vi "CO Serial CAL & Data Recording & DECADEv4.1.vi"() -> ()   [LabVIEW 2014]
uses:
  <vilib>/Platform/TimedLoop/XDataNode/timing_clust.ctl
  <vilib>/Platform/TimedLoop/XDataNode/nitl_modes.ctl
  <vilib>/Platform/TimedLoop/XDataNode/wakeup.ctl
  C:/Program Files (x86)/National Instruments/LabVIEW 2014/examples/Data Communication/Network Streams/Simple Network Streams/support/Network Stream Command.ctl
  <vilib>/Utility/error.llb/whitespace.ctl
  <vilib>/Instr/_visa.llb/VISA Configure Serial Port (Instr).vi
  <vilib>/Utility/tcp.llb/UDP Multicast Write-Only Open.vi
  <vilib>/platform/TimedLoop/XDataNode/XDataNode.xnode
  <vilib>/Platform/TimedLoop/XDataNode/XDNodeRunTimeDep.lvlib
panel:
  out "Stop File Write":bool
  out "Default file name":string
  in  "Flight Number 2":string="XXXX"
  out "status":bool
  out "CO Vacuum":bool
  out "CO CAL":bool
  out "error out":errorcluster
  out "CO Vacuum?":i16
  out "Control data":i32[](array[numeric])
  out "Control data out":string
  in  "VISA resource name":refnum<visa-resource-name>="ASRL8::INSTR"
  out "Serial VISA error":errorcluster
  out "SEPTIC TCP Error Out":errorcluster
  out "TCP packet\nSend To SEPTIC":bool
  in  "msec to wait":u32=330 caption="mSec to Wait"
  out "UDP Time Stamp Offset":i32=1
  out "Scan from String Error \nCounter from process loop":i32
  out "TCP Binary Packet":string
  in  "ue9LJ temp":u16
  out "FISH TCP Error Out":errorcluster
  out "TCP packet\nSend To FISH":bool
  out "UDP_Out_Error Out":errorcluster
  out "Data Array":string[](array[string])
  out "UDP_Out Status":bool
  out "Data Process Status":bool
  out "Command In":string[](array[string])
  out "ERR Counter":i32
  out "UDP_Out":string
  out "UDP_Pack_num":u32
  out "Flight Number":string
  out "OK RAW COUNTER":i32
  out "IN_CAL?":bool
  out "Redundent DATA":string
  out "Data String":string
  out "CO_Data_Buffer":string[](array[string])
  out "RAW DATA":string
  out "loop count":i32
  out "Number of Read error":i32
  out "Command In":string
  # "Pre-flight"
  # "CONC"
  # "SIG"
  # "SENS"
  # "ZERO"
  # "Lamp flow controller"
  # "Lamp temperature"
  # "Monochromater flow controller"
  # "Monochromater temperature"
  # "Monochromater pressure"
  # "Fluorescence cell pressure"
  # "Calibration gas pressure"
  # "Cell temperature"
  # "Calibration Concentration"
  # "ERROR number"
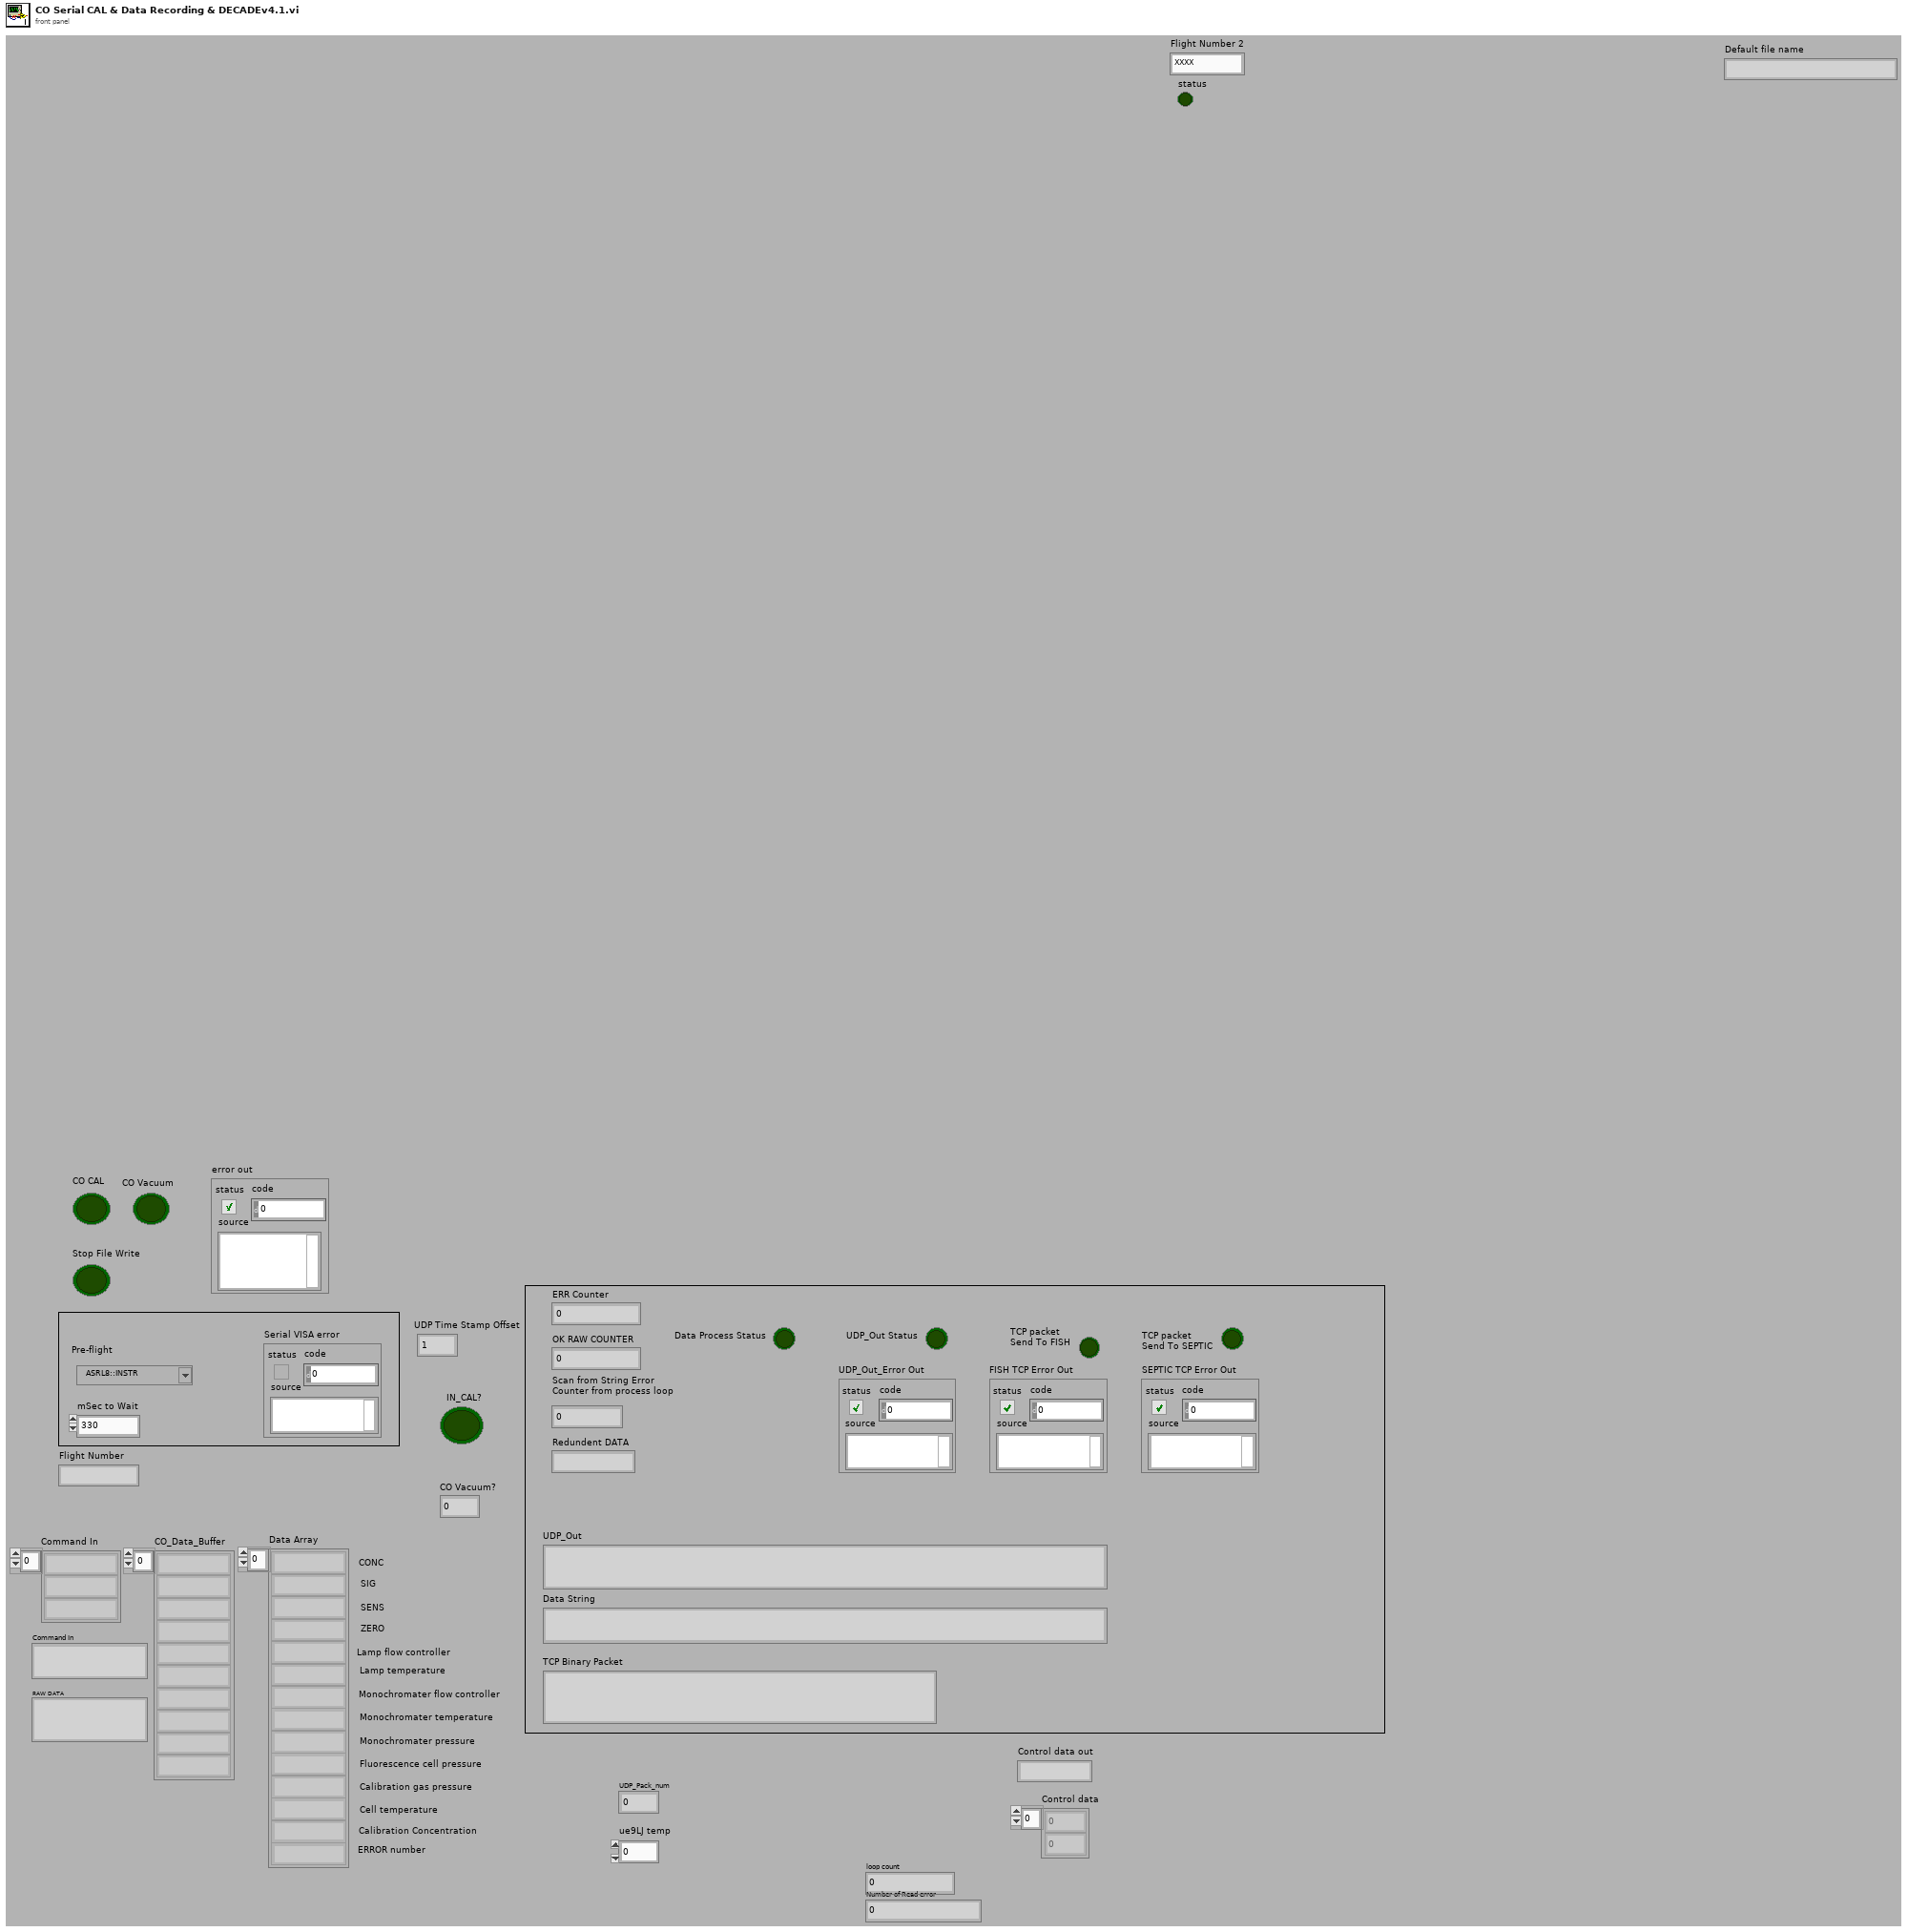
[diagram p1: front panel]
types:
  T1 = typedef "XDNodeRunTimeDep.lvlib/timing_clust.ctl" = cluster{"Expected End [f-1]":u64, "Actual End [f-1]":u64, "Finished Late? [f-1]":bool, "Expected End [i-1]":u64, "Actual End [i-1]":u64, "Finished Late? [i-1]":bool, "Expected Start [i]":u64, "Actual Start [i]":u64, "Expected Start [f]":u64, "Actual Start [f]":u64, "Source Name":string, "Structure Name":string, "Period":i64, "Deadline":i64, "Offset":i64, "Start":i64, "Priority":i32, "Timeout":i32, "Mode":T2, "Wakeup Reason":T3, "Error":errorcluster, "Source Type":string, "Secondary Source Type":string, "Global End Time":u64, "Global Start Time":u64, "Frame Duration":u64, "Iteration Duration":u64, "Assigned CPU":i32, "I/O Scan Engine Mode":u32}
  T2 = typedef "XDNodeRunTimeDep.lvlib/nitl_modes.ctl" = enum32{"No Change", "Process missed periods, maintain original phase", "Discard missed periods, maintain original phase", "Process missed periods, ignore original phase", "Discard missed periods, ignore original phase"}
  T3 = typedef "XDNodeRunTimeDep.lvlib/wakeup.ctl" = enum32{"Normal", "Aborted", "Asynchronous wakeup", "Timing source error", "Timed loop error", "Timeout"}
  T4 = typedef "Network Stream Command.ctl" = cluster{"Message":string, "Message Data":variant}
  T5 = enum16{"open", "replace", "create", "open or create", "replace or create", "replace or create with confirmation"}
  T6 = typedef "whitespace.ctl" = u16
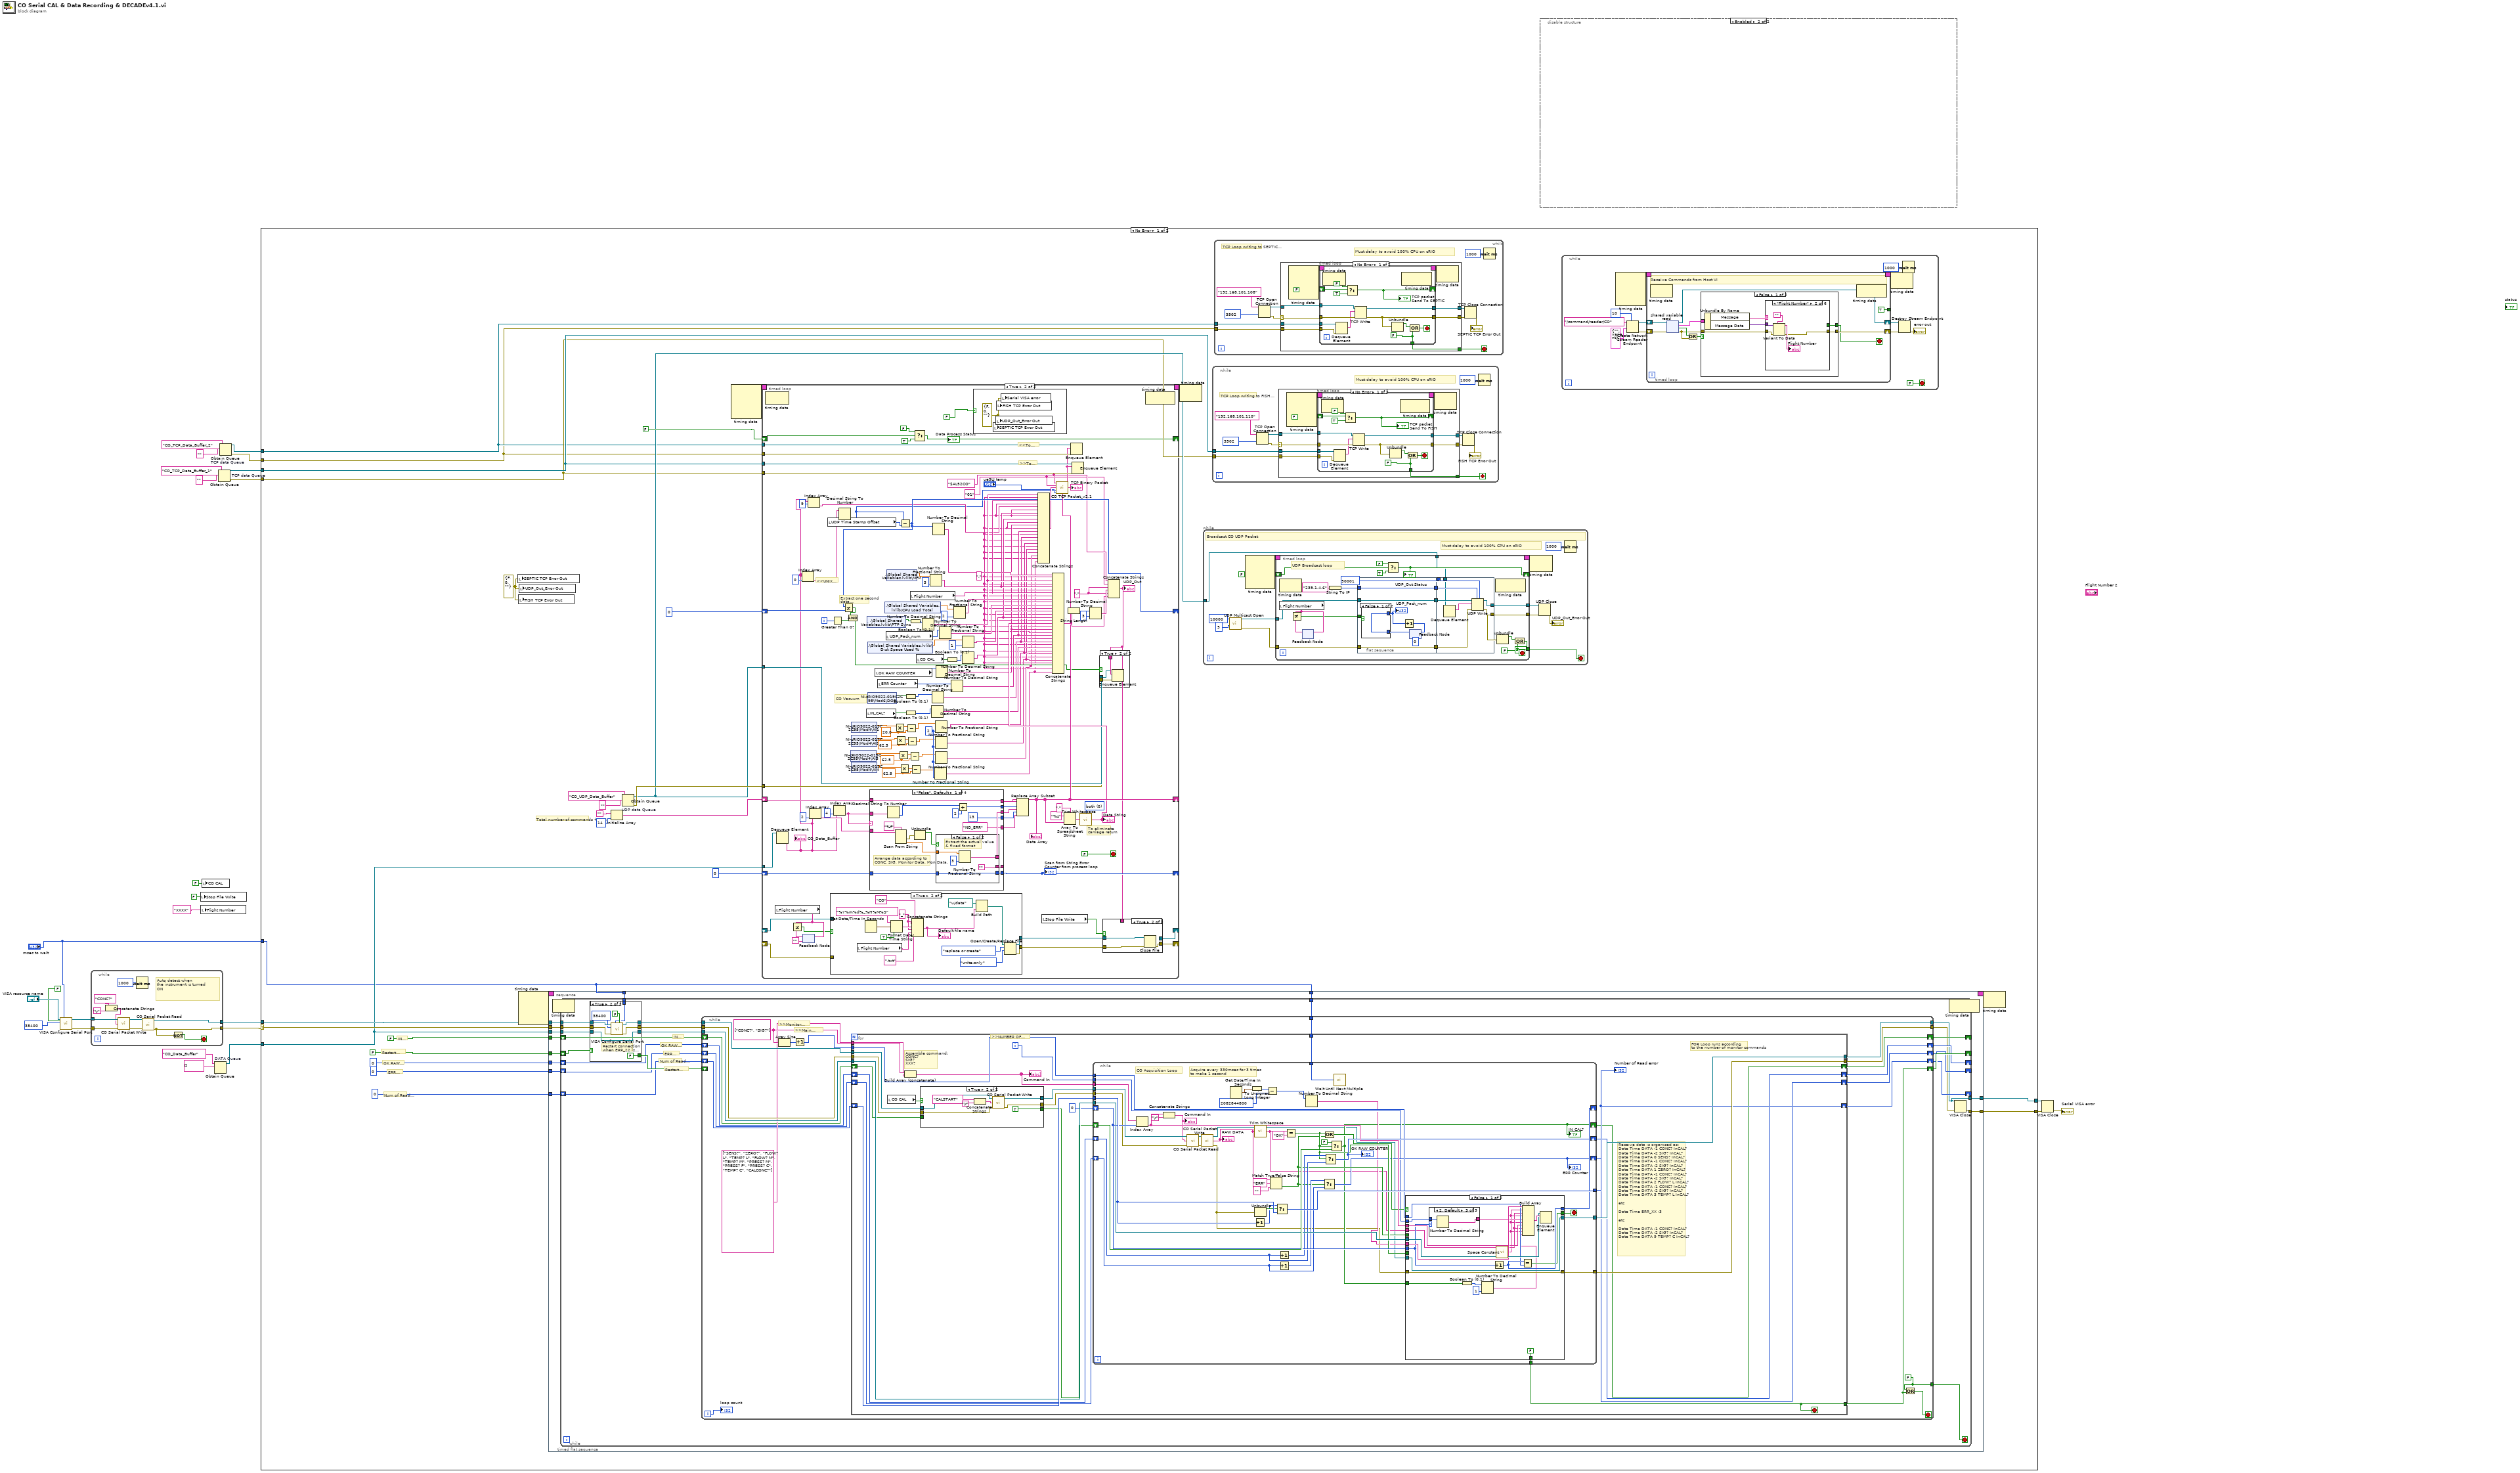
[diagram p0: block diagram]
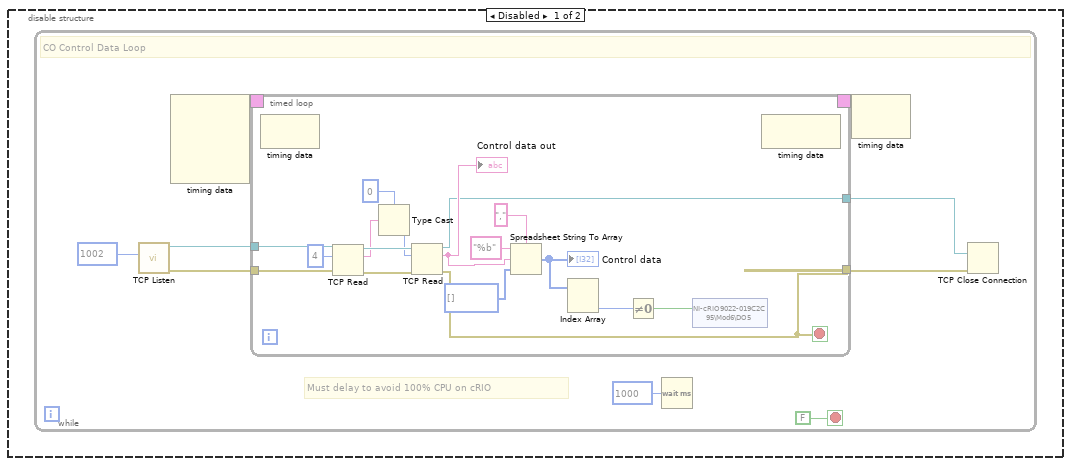
[diagram p2: hidden frame]
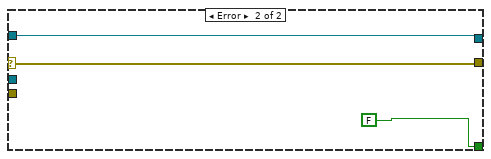
[diagram p3: hidden frame]
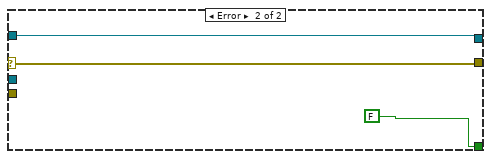
[diagram p4: hidden frame]
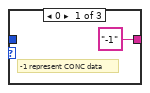
[diagram p6: hidden frame]
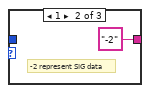
[diagram p7: hidden frame]
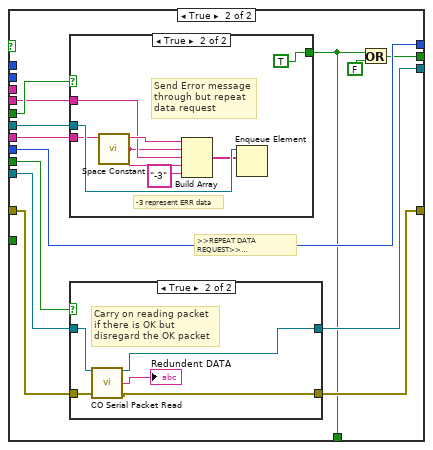
[diagram p8: hidden frame]
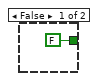
[diagram p10: hidden frame]
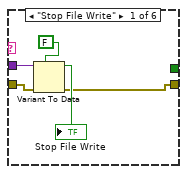
[diagram p12: hidden frame]
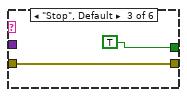
[diagram p13: hidden frame]
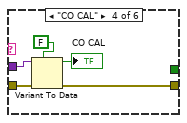
[diagram p14: hidden frame]
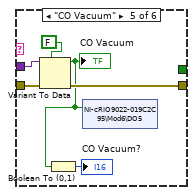
[diagram p15: hidden frame]
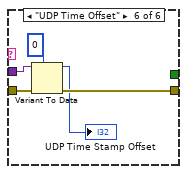
[diagram p16: hidden frame]
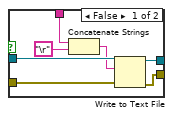
[diagram p19: hidden frame]
diagram:
  n1 = call-poly "VISA Configure Serial Port"("VISA resource name"="VISA resource name", "timeout (10sec)"="msec to wait", "Enable Termination\nChar (T)"=FALSE ("Enable Termination\nChar (T)"), "baud rate (9600)"=u32 38400) -> ("VISA resource name out"=w12:refnum<visa-resource-name>, "error out"=w11:errorcluster)  [unwired: 10 in]
  n2 = while {
    tunnel: w12 -> [w36]
    tunnel: w11 -> [w35]
    tunnel: [w29] -> w10
    tunnel: [w30] -> w9
    stop <- w34 stop-if-true
    # "Auto detect when\nthe instrument is turned \nON"
    n3 = Concatenate Strings("CONC?" ("Data in"), "\r") -> (w26:string)
    n4 = call "CO Serial Packet Write.vi"("VISA resource name In"=w36, "Data in"=w26, "error in (no error)"=w35) -> ("VISA resource name Out"=w32:refnum<visa-resource-name>, "error out"=w31:errorcluster)  [unwired: 11 in]
    n5 = Wait (ms)(milliseconds to wait=u32 1000) -> ()  [unwired: 1 out]
    n6 = call "CO Serial Packet Read.vi"("VISA resource In"=w32, "error in"=w31) -> ("VISA resource Out"=w29:refnum<visa-resource-name>, "error out"=w30:errorcluster)  [unwired: 11 in, 1 out]
    n7 = Not(x=w30) -> (.not. x?=w34:bool)
  }
  n8 = local write "Stop File Write"(FALSE ("Stop File Write")) -> ()
  n9 = local write "Flight Number"("XXXX" ("Flight Number")) -> ()
  n10 = local write "CO CAL"(FALSE ("CO CAL")) -> ()
  n11 = Obtain Queue "DATA Queue"(name (unnamed)="CO_Data_Buffer", element data type=string[] []) -> (queue out=w23:refnum<queue>)  [unwired: 3 in, 2 out]
  n12 = Obtain Queue "TCP data Queue"(name (unnamed)="CO_TCP_Data_Buffer_1", element data type="") -> (queue out=w22:refnum<queue>, error out=w21:errorcluster)  [unwired: 3 in, 1 out]
  n13 = Obtain Queue "TCP data Queue"(name (unnamed)="CO_TCP_Data_Buffer_2", element data type="") -> (queue out=w20:refnum<queue>, error out=w19:errorcluster)  [unwired: 3 in, 1 out]
  n14 = case shown="No Error" w9 {
    selector: w9 -> [w64 w715]
    tunnel: w10 -> [w65 w714]
    tunnel: [w66 w715] -> w15
    tunnel: [w42 w714] -> w14
    tunnel: w23 -> [w63 _]
    tunnel: w22 -> [w52 _]
    tunnel: w21 -> [w51 _]
    tunnel: w20 -> [w50 _]
    tunnel: w19 -> [w49 _]
    tunnel: "msec to wait" -> [w37 _]
    frame No Error {
      w48 = errorcluster {"status"=FALSE, "code"=0, "source"=""} ("UDP_Out_Error Out")
      # "Restart connection?"
      # "IN CAL?"
      # "OK RAW Counter"
      # "ERR Counter"
      # "Num of Read Error"
      # "Total number of commands + ERR"
      n15 = local write "SEPTIC TCP Error Out"(w48) -> ()
      n16 = node-c288() -> (w39:T1)  [unwired: 4 in]
      n17 = local write "FISH TCP Error Out"(w48) -> ()
      n18 = local write "UDP_Out_Error Out"(w48) -> ()
      n19 = timed-sequence {
        timing: w39 -> [_]
        timing-out: [_] -> w38
        tunnel: [w162] -> w66
        tunnel: w65 -> [w161]
        tunnel: w64 -> [w160]
        tunnel: w63 -> [w159]
        tunnel: FALSE -> [w158]
        tunnel: 0 -> [w157]
        tunnel: 0 -> [w156]
        tunnel: 0 -> [w155]
        tunnel: FALSE ("IN_CAL?") -> [w154]
        tunnel: [w153] -> w42
        tunnel: w37 -> [w152]
        tunnel: w37 -> [w151]
        n20 = timed-flat-sequence {
          tunnel: [w174] -> w162
          tunnel: w161 -> [w173]
          tunnel: w160 -> [w172]
          tunnel: w159 -> [w171]
          tunnel: w158 -> [w170]
          tunnel: w157 -> [w169]
          tunnel: w156 -> [w168]
          tunnel: w155 -> [w167]
          tunnel: w154 -> [w166]
          tunnel: [w165] -> w153
          tunnel: w152 -> [w164]
          tunnel: w151 -> [w163]
          n21 = node-c288() -> ()  [unwired: 1 in, 1 out]
          n22 = while {
            tunnel: [w179] -> w174
            tunnel: w173 -> [w196]
            tunnel: w172 -> [w195]
            tunnel: w171 -> [w193]
            shift-right: [w190] -> _
            shift-left: w170 -> [w191]
            shift-right: [w186] -> _
            shift-left: w169 -> [w187]
            shift-right: [w183] -> _
            shift-left: w168 -> [w185]
            shift-right: [w182] -> _
            shift-left: w167 -> [w184]
            shift-right: [w180] -> _
            shift-left: w166 -> [w181]
            tunnel: [w177] -> w165
            tunnel: w164 -> [w176]
            tunnel: w163 -> [w175]
            stop <- w189 stop-if-true
            # "Restart connection?"
            # "Num of Read Error"
            # "ERR Counter"
            # "IN CAL?"
            # "OK RAW Counter"
            n23 = case shown="True" w191 {
              selector: w191 -> [w198 _]
              tunnel: [w201 w207] -> w197
              tunnel: w196 -> [w201 w208]
              tunnel: [w200 w206] -> w194
              tunnel: w195 -> [w200 w205]
              tunnel: [w199 w210] -> w192
              tunnel: w193 -> [w199 w210]
              tunnel: [w198 FALSE] -> w188
              tunnel: w175 -> [_ w202]
              frame False {
              }
              frame True {
                # "Restart connection\nwhen ERR_22 is detected"
                n24 = call-poly "VISA Configure Serial Port"("VISA resource name"=w208, "timeout (10sec)"=w202, "Enable Termination\nChar (T)"=FALSE ("Enable Termination\nChar (T)"), "baud rate (9600)"=u32 38400, "error in (no error)"=w205) -> ("VISA resource name out"=w207:refnum<visa-resource-name>, "error out"=w206:errorcluster)  [unwired: 9 in]
              }
            }
            n25 = while {
              tunnel: [w232] -> w178
              tunnel: w197 -> [w231]
              tunnel: w194 -> [w230]
              tunnel: [w229] -> w177
              tunnel: w192 -> [w228]
              shift-right: [w219] -> w186
              shift-left: w187 -> [w223]
              shift-right: [w218] -> w183
              shift-left: w185 -> [w222]
              shift-right: [w217] -> w180
              shift-left: w181 -> [w221]
              shift-right: [w216] -> w182
              shift-left: w184 -> [w220]
              tunnel: [w212] -> w189
              shift-right: [w213] -> w190
              shift-left: w188 -> [_]
              tunnel: w176 -> [w211]
              i -> [w215]
              stop <- w214 stop-if-true
              w212 = FALSE
              w227 = string[] ["CONC?", "SIG?"]
              # ">>Main commands>>"
              # ">>Monitor Command>>"
              n26 = Array Size(array=w227) -> (size(s)=w224:i32)
              n27 = Increment(x=w224) -> (x+1=w226:i32)
              n28 = for {
                tunnel: w231 -> [w252]
                tunnel: w230 -> [w251]
                tunnel: [w257] -> w232
                shift-right: [w255] -> w216
                shift-left: w220 -> [w256]
                tunnel: [w254] -> w229
                tunnel: w228 -> [w253]
                tunnel: w226 -> [w247]
                shift-right: [w245] -> w217
                shift-left: w221 -> [w246]
                shift-right: [w243] -> w218
                shift-left: w222 -> [w244]
                shift-right: [w241] -> w219
                shift-left: w223 -> [w242]
                tunnel: string[] ["SENS?", "ZERO?", "FLOW? L", "TEMP? L", "FLOW? M", "TEMP? M", "PRESS? M", "PRESS? F", "PRESS? C", "TEMP? C", "CALCONC?"] -> [w238] mode=indexing
                tunnel: w227 -> [w239]
                tunnel: [w236] -> w213
                tunnel: w211 -> [w234]
                i -> [w237]
                stop <- w236 stop-if-true
                # "Receive data is organised as:\nDate Time DATA -1 CONC? InCAL?\nDate Time DATA -2 SIG? InCAL?\nDate Time DATA 0 SENS? InCAL?\nDate Time DATA -1 CONC? InCAL?\nDate Time DATA -2 SIG? InCAL?\nDate Time DATA 1 ZERO? InCAL?\nDate Time DATA -1 CONC? InCAL?\nDate Time DATA -2 SIG? InCAL?\nDate Time DATA 2 FLOW? L InCAL?\nDate Time DATA -1 CONC? InCAL?\nDate Time DATA -2 SIG? InCAL?\nDate Time DATA 3 TEMP? L InCAL?\n\netc\n\nDate Time ERR_XX -3\n\netc\n\nDate Time DATA -1 CONC? InCAL?\nDate Time DATA -2 SIG? InCAL?\nDate Time DATA 9 TEMP? C InCAL?"
                # "FOR Loop runs according\nto the number of monitor commands"
                # "Assemble command:\nCONC?\nSIG?\nXXX?"
                # ">>NUMBER OF COMMANDS>>"
                n29 = local read "CO CAL"() -> (w233:bool)
                n30 = Build Array (concatenate)(w239, w238) -> (w240:string[])
                "Command In" <- w240
                n31 = case shown="True" w233 {
                  tunnel: w252 -> [w357 w359]
                  tunnel: w251 -> [w356 w362]
                  tunnel: [w357 w360] -> w250
                  tunnel: [w356 w361] -> w249
                  tunnel: [w355 TRUE ("IN_CAL?")] -> w248
                  tunnel: w246 -> [w355 _]
                  frame False {
                  }
                  frame True {
                    n32 = Concatenate Strings("CALSTART" ("string"), "\r") -> (w358:string)
                    n33 = call "CO Serial Packet Write.vi"("VISA resource name In"=w359, "Data in"=w358, "error in (no error)"=w362) -> ("VISA resource name Out"=w360:refnum<visa-resource-name>, "error out"=w361:errorcluster)  [unwired: 11 in]
                  }
                }
                n34 = while {
                  tunnel: w249 -> [w264]
                  tunnel: [w291] -> w257
                  tunnel: w256 -> [w303]
                  tunnel: [w302] -> w255
                  tunnel: w240 -> [w295]
                  tunnel: [w292] -> w254
                  tunnel: w253 -> [w290]
                  tunnel: w250 -> [w266]
                  shift-right: [w267] -> w245
                  shift-left: w248 -> [w297]
                  shift-right: [w294] -> _
                  shift-left: 0 -> [w296]
                  tunnel: w247 -> [w287]
                  shift-right: [w284] -> w243
                  shift-left: w244 -> [w285]
                  shift-right: [w278] -> w241
                  shift-left: w242 -> [w280]
                  tunnel: w237 -> [w277]
                  tunnel: [w272] -> w236
                  tunnel: w234 -> [w258]
                  stop <- w293 stop-if-true
                  # "Acquire every 330msec for 3 times\nto make 1 second"
                  # "CO Acquisition Loop"
                  n35 = Index Array(array=w295, index=w296) -> (element=w289:string)
                  n36 = Concatenate Strings(w289, "\r") -> (w265:string)
                  "Command In" <- w265
                  n37 = call "CO Serial Packet Write.vi"("VISA resource name In"=w266, "Data in"=w265, "error in (no error)"=w264) -> ("VISA resource name Out"=w262:refnum<visa-resource-name>, "error out"=w263:errorcluster)  [unwired: 11 in]
                  n38 = call "CO Serial Packet Read.vi"("VISA resource In"=w262, "error in"=w263) -> ("VISA resource Out"=w261:refnum<visa-resource-name>, "Data Out"=w259:string, "error out"=w260:errorcluster)  [unwired: 11 in]
                  "RAW DATA" <- w259
                  n39 = Get Date/Time In Seconds() -> (seconds since 1Jan1904=w273:timestamp)
                  n40 = To Unsigned Long Integer(number=w273) -> (unsigned 32bit integer=w276:u32)
                  n41 = Increment(x=w303) -> (x+1=w299:i32)
                  n42 = call <vilib>:"Trim Whitespace.vi"("string"=w259) -> ("trimmed string"=w271:string)  [unwired: 1 in]
                  n43 = Unbundle(w260) -> ("status"=w300:bool)  [unwired: 2 out]
                  n44 = Subtract(x=w276, y=u32 2082844800) -> (x-y=w268:u32)
                  n45 = Match True/False String(2:"" ("false string"), 3:"ERR" ("true string"), 4:w259) -> (0:w279:bool)  [unwired: 1 out]
                  n46 = Select(t=w299, s=w300, f=w303) -> (s? t:f=w302:i32)
                  n47 = Increment(x=w285) -> (x+1=w286:i32)
                  n48 = Increment(x=w280) -> (x+1=w281:i32)
                  n49 = Equal?(x=w271, y="OK" ("string")) -> (x = y?=w282:bool)
                  n50 = Number To Decimal String(number=w268) -> (decimal integer string=w274:string)  [unwired: 1 in]
                  n51 = Select(t=w281, s=w279, f=w280) -> (s? t:f=w278:i32)
                  "ERR Counter" <- w278
                  n52 = Select(t=w286, s=w282, f=w285) -> (s? t:f=w284:i32)
                  "OK RAW COUNTER" <- w284
                  n53 = Compound Arithmetic op=OR(w282, w279) -> (w283:bool)
                  n54 = Select(t=FALSE, s=w282, f=w297) -> (s? t:f=w267:bool)
                  "IN_CAL?" <- w267
                  n55 = call "Wait Until Next Multiple"("Count(mSec)"=w258) -> ()  [unwired: 1 out]
                  n56 = case shown="False" w283 {
                    tunnel: w296 -> [w311 w339]
                    tunnel: [w322 w339] -> w294
                    tunnel: [w316 w329] -> w293
                    tunnel: w261 -> [w321 w338]
                    tunnel: w260 -> [w320 w337]
                    tunnel: [w321 w336] -> w292
                    tunnel: [w320 w335] -> w291
                    tunnel: w290 -> [w318 w333]
                    tunnel: w271 -> [w309 w331]
                    tunnel: w289 -> [w312 _]
                    tunnel: w274 -> [w317 w332]
                    tunnel: w279 -> [_ w334]
                    tunnel: w287 -> [w315 _]
                    tunnel: w282 -> [_ w330]
                    tunnel: w277 -> [w314 _]
                    tunnel: [FALSE w327] -> w272
                    tunnel: w267 -> [w308 _]
                    frame False {
                      n57 = case shown="2, Default" w311 {
                        tunnel: w314 -> [_ _ w326]
                        tunnel: ["-1" "-2" w325] -> w313
                        frame 0 {
                          # "-1 represent CONC data"
                        }
                        frame 1 {
                          # "-2 represent SIG data"
                        }
                        frame 2, Default {
                          n58 = Number To Decimal String(number=w326) -> (decimal integer string=w325:string)  [unwired: 1 in]
                        }
                      }
                      n59 = Boolean To (0,1)(Boolean=w308) -> (0, 1=w307:i16)
                      n60 = Number To Decimal String(number=w307, width (-)=i16 1) -> (decimal integer string=w304:string)
                      n61 = Increment(x=w311) -> (x+1=w322:i32)
                      n62 = call <vilib>:"Space Constant.vi"() -> ("String"=w305:string)
                      n63 = Equal?(x=w322, y=w315) -> (x = y?=w316:bool)
                      n64 = Build Array(w317, w305, w309, w305, w313, w305, w312, w309, w305, w304) -> (w319:string[])
                      n65 = Enqueue Element(queue=w318, element=w319) -> ()  [unwired: 2 in, 3 out]
                    }
                    frame True {
                      # ">>REPEAT DATA REQUEST>>\nif OK or ERR"
                      n66 = case shown="True" w334 {
                        tunnel: w333 -> [_ w354]
                        tunnel: w332 -> [_ w352]
                        tunnel: w331 -> [_ w351]
                        tunnel: [FALSE TRUE] -> w327
                        frame False {
                        }
                        frame True {
                          # "-3 represent ERR data"
                          # "Send Error message\nthrough but repeat\ndata request"
                          n67 = call <vilib>:"Space Constant.vi"() -> ("String"=w350:string)
                          n68 = Build Array(w352, w350, w351, w350, "-3" ("element")) -> (w353:string[])
                          n69 = Enqueue Element(queue=w354, element=w353) -> ()  [unwired: 2 in, 3 out]
                        }
                      }
                      n70 = case shown="True" w330 {
                        tunnel: w338 -> [w340 w345]
                        tunnel: w337 -> [w341 w346]
                        tunnel: [w340 w344] -> w336
                        tunnel: [w341 w342] -> w335
                        frame False {
                        }
                        frame True {
                          # "Carry on reading packet\nif there is OK but\ndisregard the OK packet"
                          n71 = call "CO Serial Packet Read.vi"("VISA resource In"=w345, "error in"=w346) -> ("VISA resource Out"=w344:refnum<visa-resource-name>, "Data Out"=→"Redundent DATA":string, "error out"=w342:errorcluster)  [unwired: 11 in]
                        }
                      }
                      n72 = Or(x=w327, y=FALSE) -> (x .or. y?=w329:bool)
                    }
                  }
                }
                "Number of Read error" <- w255
              }
              n73 = Or(x=w212, y=w213) -> (x .or. y?=w214:bool)
              "loop count" <- w215
            }
            n74 = VISA Close(VISA resource name=w177, error in (no error)=w178) -> (error out=w179:errorcluster)
          }
          n75 = node-c288() -> ()  [unwired: 1 in, 1 out]
        }
      }
      n76 = Initialize Array("", 14) -> (w60:string[])
      n77 = Obtain Queue "UDP data Queue"(name (unnamed)="CO_UDP_Data_Buffer", element data type="") -> (queue out=w55:refnum<queue>, error out=w56:errorcluster)  [unwired: 3 in, 1 out]
      n78 = node-c288() -> (w41:T1)  [unwired: 4 in]
      n79 = timed-loop {
        tunnel: w63 -> [w548]
        shift-right: [w523] -> _
        shift-left: w60 -> [w537]
        shift-right: [w524] -> _
        shift-left: FALSE -> [w527]
        tunnel: w52 -> [w522]
        tunnel: w51 -> [w521]
        tunnel: w55 -> [w519]
        tunnel: w56 -> [w518]
        shift-right: [w516] -> _
        shift-left: 0 -> [w517]
        shift-right: [w504] -> _
        shift-left: 0 -> [w510]
        tunnel: w50 -> [w508]
        tunnel: w49 -> [w507]
        timing: w41 -> [_]
        timing-out: [_] -> w40
        shift-right: [w495] -> _
        shift-left: _ -> [w488]
        shift-right: [w486] -> _
        shift-left: _ -> [w487]
        i -> [w513]
        stop <- FALSE stop-if-true
        w469 = 62.5 ("y")
        w470 = 62.5 ("y")
        w473 = 62.5 ("y")
        w476 = 20.0 ("y")
        w498 = i16 2 ("precision (6)")
        w529 = T6 0 items=["both", "start of string", "end of string"] ("location (both)")
        w438 = ","
        w434 = "01"
        w540 = ","
        w435 = "$AL52CO"
        # "CO Vacuum"
        # ">>To SEPTIC>>"
        # ">>To FISH>>"
        # "Extract one second data\nfor UDP sending"
        # ">>UNIX TIME>>"
        # "To eliminate\ncarriage return"
        n80 = node-c288() -> ()  [unwired: 1 in, 1 out]
        n81 = local read "Flight Number"() -> (w493:string)
        n82 = Dequeue Element(queue=w548) -> (element=w500:string[])  [unwired: 2 in, 3 out]
        "CO_Data_Buffer" <- w500
        n83 = Index Array(array=w500, index=0) -> (element=w511:string)
        n84 = feedback #1("" ("Flight Number")) -> (w492:string)
        n85 = Not Equal?(x=w493, y=w492) -> (x != y?=w491:bool)
        n86 = feedback-in #1(w493) -> ()
        n87 = Index Array(array=w500, index=9) -> (element=w447:string)
        n88 = Index Array(array=w500, index=2) -> (element=w535:string)
        n89 = local read "UDP Time Stamp Offset"() -> (w450:i32)
        n90 = case shown="True" w491 {
          tunnel: [w550 w552] -> w490
          tunnel: [w549 w551] -> w489
          tunnel: w488 -> [w550 _]
          tunnel: w487 -> [w549 _]
          frame False {
          }
          frame True {
            w559 = "_" ("string")
            n91 = local read "Flight Number"() -> (w565:string)
            n92 = Get Date/Time In Seconds() -> (seconds since 1Jan1904=w560:timestamp)
            n93 = Format Date/Time String(time format string (%c)="%Y%m%d%_%H%M%S", seconds (now)=w560, UTC format=TRUE) -> (date/time string=w563:string)
            n94 = Concatenate Strings("CO" ("string"), w559, w563, w559, w565, ".txt" ("string")) -> (w557:string)
            "Default file name" <- w557
            n95 = Build Path(base path=path "u:/data", name or relative path=w557) -> (appended path=w553:path)
            n96 = Open/Create/Replace File(file path (use dialog)=w553, operation (0:open)=T5."replace or create", access (0:read/write)=enum16{"read/write", "read-only", "write-only"}."write-only") -> (refnum out=w552:refnum<file>, error out=w551:errorcluster)  [unwired: 3 in, 1 out]
          }
        }
        n97 = Greater Than 0?(x=w513) -> (x > 0?=w512:bool)
        n98 = Index Array(array=w500, index=4) -> (element=w536:string)
        n99 = Decimal String To Number(string=w511) -> (number=w433:i32)  [unwired: 2 in, 1 out]
        n100 = shared-variable "NI-cRIO9022-019C2C95\\Mod4\\AI3"() -> (w468:dbl)  [unwired: 1 in, 1 out]
        n101 = shared-variable "NI-cRIO9022-019C2C95\\Mod4\\AI4"() -> (w466:dbl)  [unwired: 1 in, 1 out]
        n102 = shared-variable "NI-cRIO9022-019C2C95\\Mod4\\AI1"() -> (w478:dbl)  [unwired: 1 in, 1 out]
        n103 = shared-variable "NI-cRIO9022-019C2C95\\Mod4\\AI2"() -> (w472:dbl)  [unwired: 1 in, 1 out]
        n104 = local read "IN_CAL?"() -> (w455:bool)
        n105 = shared-variable ".\\Global Shared Variables.lvlib\\PTP Sync"() -> (w479:bool)  [unwired: 1 in, 1 out]
        n106 = shared-variable ".\\Global Shared Variables.lvlib\\Disk Space Used %"() -> (w459:dbl)  [unwired: 1 in, 1 out]
        n107 = shared-variable "NI-cRIO9022-019C2C95\\Mod6\\DO5"() -> (w452:bool)  [unwired: 1 in, 1 out]
        n108 = case shown="\"False\", Default" w536 {
          tunnel: w536 -> [w596 _ _ _]
          tunnel: w537 -> [w597 w619 w641 w655]
          tunnel: w535 -> [w588 w613 w635 w651]
          tunnel: [w597 w619 w641 w655] -> w534
          tunnel: [w594 0 ("index") 1 ("index") w652] -> w533
          tunnel: [w587 w609 w631 w651] -> w532
          tunnel: [w586 w610 w632 ""] -> _
          tunnel: w517 -> [w585 w612 w634 w653]
          tunnel: [w584 w611 w633 w653] -> w516
          tunnel: [13 ("index") 13 ("index") 13 ("index") w652] -> w503
          tunnel: ["NO_ERR" "NO_ERR" "NO_ERR" w651] -> w502
          frame "False", Default {
            # "Arrange data according to\nCONC, SIG, Monitor Data, Mon Data,"
            n109 = Decimal String To Number(string=w596) -> (number=w593:i32)  [unwired: 2 in, 1 out]
            n110 = Scan From String(format string="%f", input string=w588) -> (error out=w590:errorcluster, output 1=w591:dbl)  [unwired: 3 in, 2 out]
            n111 = Unbundle(w590) -> ("status"=w589:bool)  [unwired: 2 out]
            n112 = case shown="False" w589 {
              tunnel: [w602 ""] -> w587
              tunnel: w591 -> [w601 _]
              tunnel: w585 -> [w600 w605]
              tunnel: [w600 w604] -> w584
              tunnel: ["" "Scan from string error"] -> w586
              frame False {
                # "Extract the actual value\n& fixed format"
                n113 = Number To Fractional String(number=w601, precision (6)=i16 3) -> (F-format string=w602:string)  [unwired: 2 in]
              }
              frame True {
                # "If scan from string error,\nreplace data with empty\nstring"
                n114 = Increment(x=w605) -> (x+1=w604:i32)
              }
            }
            n115 = Add(x=w593, y=2) -> (x+y=w594:i32)
          }
          frame "-1" {
            # "Arrange data according to\nCONC, SIG, Monitor Data, Mon Data,"
            # "-1 represent CONC data"
            n116 = Scan From String(format string="%f", input string=w613) -> (error out=w615:errorcluster, output 1=w616:dbl)  [unwired: 3 in, 2 out]
            n117 = Unbundle(w615) -> ("status"=w614:bool)  [unwired: 2 out]
            n118 = case shown="False" w614 {
              tunnel: [w624 ""] -> w609
              tunnel: w616 -> [w623 _]
              tunnel: w612 -> [w622 w627]
              tunnel: [w622 w626] -> w611
              tunnel: ["" "Scan from string error"] -> w610
              frame False {
                # "Extract the actual value\n& fixed format"
                n119 = Number To Fractional String(number=w623, precision (6)=i16 5) -> (F-format string=w624:string)  [unwired: 2 in]
              }
              frame True {
                # "If scan from string error,\nreplace data with empty\nstring"
                n120 = Increment(x=w627) -> (x+1=w626:i32)
              }
            }
          }
          frame "-2" {
            # "Arrange data according to\nCONC, SIG, Monitor Data, Mon Data,"
            # "-2 represent SIG data"
            n121 = Scan From String(format string="%f", input string=w635) -> (error out=w637:errorcluster, output 1=w638:dbl)  [unwired: 3 in, 2 out]
            n122 = Unbundle(w637) -> ("status"=w636:bool)  [unwired: 2 out]
            n123 = case shown="False" w636 {
              tunnel: [w646 ""] -> w631
              tunnel: w638 -> [w645 _]
              tunnel: w634 -> [w644 w649]
              tunnel: [w644 w648] -> w633
              tunnel: ["" "Scan from string error"] -> w632
              frame False {
                # "Extract the actual value\n& fixed format"
                n124 = Number To Fractional String(number=w645, precision (6)=i16 3) -> (F-format string=w646:string)  [unwired: 2 in]
              }
              frame True {
                # "If scan from string error,\nreplace data with empty\nstring"
                n125 = Increment(x=w649) -> (x+1=w648:i32)
              }
            }
          }
          frame "-3" {
            w652 = 13 ("index")
            # "-3 represent ERR data"
          }
        }
        "Scan from String Error \nCounter from process loop" <- w516
        n126 = local read "OK RAW COUNTER"() -> (w538:i32)
        n127 = local read "ERR Counter"() -> (w497:i32)
        n128 = shared-variable ".\\Global Shared Variables.lvlib\\CPU Load Total"() -> (w484:dbl)  [unwired: 1 in, 1 out]
        n129 = local read "UDP_Pack_num"() -> (w544:u32)
        n130 = shared-variable ".\\Global Shared Variables.lvlib\\MFM"() -> (w483:dbl)  [unwired: 1 in, 1 out]
        n131 = Multiply(x=w478, y=w476) -> (x*y=w477:dbl)
        n132 = Multiply(x=w472, y=w473) -> (x*y=w474:dbl)
        n133 = Multiply(x=w468, y=w470) -> (x*y=w467:dbl)
        n134 = Multiply(x=w466, y=w469) -> (x*y=w465:dbl)
        n135 = Subtract(x=w433, y=w450) -> (x-y=w504:i32)
        n136 = Not Equal?(x=w504, y=w510) -> (x != y?=w514:bool)
        n137 = Compound Arithmetic op=AND(w514, w512) -> (w509:bool)
        n138 = Boolean To (0,1)(Boolean=w452) -> (0, 1=w451:i16)
        n139 = Boolean To (0,1)(Boolean=w455) -> (0, 1=w454:i16)
        n140 = Subtract(x=w477, y=w476) -> (x-y=w475:dbl)
        n141 = Subtract(x=w474, y=w473) -> (x-y=w471:dbl)
        n142 = Subtract(x=w467, y=w470) -> (x-y=w464:dbl)
        n143 = Boolean To (0,1)(Boolean=w479) -> (0, 1=w480:i16)
        n144 = local read "Flight Number"() -> (w448:string)
        n145 = Subtract(x=w465, y=w469) -> (x-y=w463:dbl)
        n146 = Select(t=FALSE, s=w527, f=TRUE) -> (s? t:f=w524:bool)
        "Data Process Status" <- w524
        n147 = local read "CO CAL"() -> (w457:bool)
        n148 = Number To Decimal String(number=w480) -> (decimal integer string=w449:string)  [unwired: 1 in]
        n149 = Number To Fractional String(number=w483, precision (6)=i16 3 ("width (-)")) -> (F-format string=w446:string)  [unwired: 2 in]
        n150 = Number To Decimal String(number=w454) -> (decimal integer string=w453:string)  [unwired: 1 in]
        n151 = Number To Decimal String(number=w451) -> (decimal integer string=w442:string)  [unwired: 1 in]
        n152 = Number To Decimal String(number=w504) -> (decimal integer string=w505:string)  [unwired: 1 in]
        n153 = Number To Fractional String(number=w463, precision (6)=w498) -> (F-format string=w437:string)  [unwired: 2 in]
        n154 = Number To Fractional String(number=w475, precision (6)=w498) -> (F-format string=w441:string)  [unwired: 2 in]
        n155 = Number To Fractional String(number=w471, precision (6)=w498) -> (F-format string=w440:string)  [unwired: 2 in]
        n156 = Number To Fractional String(number=w464, precision (6)=w498) -> (F-format string=w439:string)  [unwired: 2 in]
        n157 = Number To Decimal String(number=w538) -> (decimal integer string=w444:string)  [unwired: 1 in]
        n158 = Number To Decimal String(number=w544) -> (decimal integer string=w461:string)  [unwired: 1 in]
        n159 = Boolean To (0,1)(Boolean=w457) -> (0, 1=w458:i16)
        n160 = Number To Decimal String(number=w497) -> (decimal integer string=w443:string)  [unwired: 1 in]
        n161 = Number To Fractional String(number=w484, precision (6)=i16 2 ("width (-)")) -> (F-format string=w462:string)  [unwired: 2 in]
        n162 = Number To Fractional String(number=w459, precision (6)=i16 1 ("width (-)")) -> (F-format string=w456:string)  [unwired: 2 in]
        n163 = Number To Decimal String(number=w458) -> (decimal integer string=w445:string)  [unwired: 1 in]
        n164 = case shown="True" FALSE {
          frame False {
          }
          frame True {
            w578 = errorcluster {"status"=FALSE, "code"=0, "source"=""} ("UDP_Out_Error Out")
            n165 = local write "SEPTIC TCP Error Out"(w578) -> ()
            n166 = local write "UDP_Out_Error Out"(w578) -> ()
            n167 = local write "FISH TCP Error Out"(w578) -> ()
            n168 = local write "Serial VISA error"(w578) -> ()
          }
        }
        n169 = Replace Array Subset(array=w534, new element #1=w532, index #1=w533, new element #2=w502, index #2=w503) -> (w523:string[])
        "Data Array" <- w523
        n170 = Concatenate Strings(w449, w438, w448, w438, w447, w438, w446, w438, w445, w438, w444, w438, w443, w438, w442, w438, w441, w438, w440, w438, w439, w438, w437) -> (w436:string)
        n171 = local read "Stop File Write"() -> (w494:bool)
        n172 = call "CO TCP Packet_v2.1.vi"("ID"=w435, "Version"=w434, "TCP Packet Content"=w436, "utc_time"=w433, "ue9LJ temp"="ue9LJ temp", "Data Array"=w523) -> ("TCP Binary Packet"=w506:string)  [unwired: 9 in]
        "TCP Binary Packet" <- w506
        n173 = Array To Spreadsheet String(delimiter (Tab)=",", array=w523, 3:"%s" ("format string")) -> (spreadsheet string=w528:string)
        n174 = Enqueue Element(queue=w508, element=w506, error in (no error)=w507) -> ()  [unwired: 1 in, 3 out]
        n175 = Enqueue Element(queue=w522, element=w506, error in (no error)=w521) -> ()  [unwired: 1 in, 3 out]
        n176 = call <vilib>:"Trim Whitespace.vi"("string"=w528, "location (both)"=w529) -> ("trimmed string"=w520:string)
        "Data String" <- w520
        n177 = Concatenate Strings(w505, w438, w449, w438, w446, w438, w448, w438, w462, w438, w461, w438, w456, w438, w445, w438, w520, w438, w444, w438, w443, w438, w442, w438, w453, w438, w441, w438, w440, w438, w439, w438, w437) -> (w539:string)
        n178 = String Length(string=w539) -> (length=w543:i32)
        n179 = Number To Decimal String(number=w543, width (-)=i16 3) -> (decimal integer string=w541:string)
        n180 = Concatenate Strings(w435, w434, w540, w541, w540, w539) -> (w496:string)
        "UDP_Out" <- w496
        n181 = case shown="True" w509 {
          tunnel: w496 -> [_ w581]
          tunnel: w519 -> [_ w580]
          tunnel: w518 -> [_ w579]
          frame False {
          }
          frame True {
            n182 = Enqueue Element(queue=w580, element=w581, error in (no error)=w579) -> ()  [unwired: 1 in, 3 out]
          }
        }
        n183 = case shown="True" w494 {
          tunnel: w496 -> [w570 _]
          tunnel: w490 -> [w572 w575]
          tunnel: w489 -> [w571 w574]
          tunnel: [w567 _] -> w495
          tunnel: [w566 w573] -> w486
          frame False {
            n184 = Concatenate Strings(w570, "\r") -> (w568:string)
            n185 = Write to Text File(file (use dialog)=w572, text=w568, error in=w571) -> (refnum out=w567:refnum<file>, error out=w566:errorcluster)  [unwired: 2 out]
          }
          frame True {
            n186 = Close File(refnum=w575, error in=w574) -> (error out=w573:errorcluster)  [unwired: 1 out]
          }
        }
        n187 = node-c288() -> ()  [unwired: 1 in, 1 out]
      }
      n188 = node-c288(w40) -> ()  [unwired: 1 out]
      n189 = while {
        tunnel: w55 -> [w659]
        stop <- w660 stop-if-true
        # "Must delay to avoid 100% CPU on cRIO"
        # "Broadcast CO UDP Packet"
        n190 = call-poly <vilib>:"UDP Multicast Open.vi"("time-to-live (1)"=u16 5, "port"=u16 10000) -> ("error out"=w667:errorcluster, "connection ID"=w668:refnum<k16>)  [unwired: 8 in]
        n191 = node-c288() -> (w670:T1)  [unwired: 4 in]
        n192 = timed-loop {
          tunnel: w668 -> [w690]
          tunnel: w667 -> [w689]
          timing: w670 -> [_]
          timing-out: [_] -> w669
          shift-right: [w677] -> _
          shift-left: FALSE -> [w680]
          tunnel: [w676] -> w662
          tunnel: [w674] -> w661
          tunnel: [w672] -> w660
          tunnel: w659 -> [w671]
          stop <- w673 stop-if-true
          w672 = FALSE
          # "UDP Broadcast loop"
          n193 = node-c288() -> ()  [unwired: 1 in, 1 out]
          n194 = local read "Flight Number"() -> (w683:string)
          n195 = feedback-in #2(w683) -> ()
          n196 = feedback #2() -> (w682:string)  [unwired: 1 in]
          n197 = Not Equal?(x=w683, y=w682) -> (x != y?=w681:bool)
          n198 = String To IP(1:"239.1.4.6" ("name")) -> (0:w687:u32)
          n199 = flat-sequence {
            tunnel: w687 -> [w697]
            tunnel: w689 -> [w698]
            tunnel: w690 -> [w699]
            tunnel: [w699] -> w686
            tunnel: [w698] -> w685
            tunnel: [w697] -> w684
            tunnel: w681 -> [w696]
            tunnel: u16 50001 ("port or service name") -> [w709]
            tunnel: w686 -> [w708]
            tunnel: w685 -> [w707]
            tunnel: w684 -> [w706]
            tunnel: [w705] -> w676
            tunnel: [w704] -> w674
            tunnel: w671 -> [w702]
            frame #0 {
              n200 = feedback #3(u32 0) -> (w693:u32)
              n201 = case shown="False" w696 {
                tunnel: w693 -> [w700 _]
                tunnel: [w700 u32 0] -> w692
                frame False {
                }
                frame True {
                }
              }
              "UDP_Pack_num" <- w692
              n202 = Increment(x=w692) -> (x+1=w694:u32)
              n203 = feedback-in #3(w694) -> ()
            }
            frame #1 {
              n204 = Dequeue Element(queue=w702) -> (element=w703:string)  [unwired: 2 in, 3 out]
              n205 = UDP Write(address=w706, port or service name=w709, connection ID=w708, data in=w703, 8:w707) -> (error out=w704:errorcluster, 3:w705:refnum<k16>)  [unwired: 1 in]
            }
          }
          n206 = Select(t=FALSE, s=w680, f=TRUE) -> (s? t:f=w677:bool)
          "UDP_Out Status" <- w677
          n207 = node-c288() -> ()  [unwired: 1 in, 1 out]
          n208 = Unbundle(w674) -> ("status"=w675:bool)  [unwired: 2 out]
          n209 = Compound Arithmetic op=OR(w675, w672) -> (w673:bool)
        }
        n210 = node-c288(w669) -> ()  [unwired: 1 out]
        n211 = UDP Close(connection ID=w662, 8:w661) -> (error out=→"UDP_Out_Error Out":errorcluster)  [unwired: 1 out]
        n212 = Wait (ms)(milliseconds to wait=u32 1000) -> ()  [unwired: 1 out]
      }
      n213 = while {
        tunnel: w52 -> [w111]
        tunnel: w51 -> [w110]
        stop <- w114 stop-if-true
        # "Must delay to avoid 100% CPU on cRIO"
        # "TCP Loop writing to FISH Tank"
        n214 = TCP Open Connection(address="192.168.101.110", remote port or service name=u16 3502) -> (connection ID=w117:refnum<k5>, error out=w112:errorcluster)  [unwired: 3 in]
        n215 = case shown="No Error" w112 {
          selector: w112 -> [w122 w149]
          tunnel: w117 -> [w127 w150]
          tunnel: [w126 w150] -> w116
          tunnel: [w125 w149] -> w115
          tunnel: [w124 FALSE] -> w114
          tunnel: w111 -> [w121 _]
          tunnel: w110 -> [w120 _]
          frame No Error {
            n216 = node-c288() -> (w129:T1)  [unwired: 4 in]
            n217 = timed-loop {
              tunnel: w127 -> [w143]
              tunnel: w122 -> [w142]
              tunnel: [w141] -> w126
              tunnel: [w140] -> w125
              tunnel: [w130] -> w124
              shift-right: [w134] -> _
              shift-left: FALSE -> [w137]
              timing: w129 -> [_]
              timing-out: [_] -> w128
              tunnel: w121 -> [w133]
              tunnel: w120 -> [w132]
              stop <- w138 stop-if-true
              w130 = FALSE
              n218 = node-c288() -> ()  [unwired: 1 in, 1 out]
              n219 = Dequeue Element(queue=w133, error in (no error)=w132) -> (element=w131:string)  [unwired: 1 in, 3 out]
              n220 = Select(t=FALSE, s=w137, f=TRUE) -> (s? t:f=w134:bool)
              "TCP packet\nSend To FISH" <- w134
              n221 = TCP Write(connection ID=w143, data in=w131, error in (no error)=w142) -> (connection ID out=w141:refnum<k5>, error out=w140:errorcluster)  [unwired: 1 in, 1 out]
              n222 = Unbundle(w140) -> ("status"=w139:bool)  [unwired: 2 out]
              n223 = node-c288() -> ()  [unwired: 1 in, 1 out]
              n224 = Compound Arithmetic op=OR(w139, w130) -> (w138:bool)
            }
            n225 = node-c288(w128) -> ()  [unwired: 1 out]
          }
          frame Error {
          }
        }
        n226 = TCP Close Connection(connection ID=w116, error in (no error)=w115) -> (error out=→"FISH TCP Error Out":errorcluster)  [unwired: 1 in, 1 out]
        n227 = Wait (ms)(milliseconds to wait=u32 1000) -> ()  [unwired: 1 out]
      }
      n228 = while {
        tunnel: w50 -> [w69]
        tunnel: w49 -> [w68]
        stop <- w72 stop-if-true
        # "Must delay to avoid 100% CPU on cRIO"
        # "TCP Loop writing to SEPTIC Tank"
        n229 = TCP Open Connection(address="192.168.101.108", remote port or service name=u16 3502) -> (connection ID=w75:refnum<k5>, error out=w70:errorcluster)  [unwired: 3 in]
        n230 = case shown="No Error" w70 {
          selector: w70 -> [w80 w107]
          tunnel: w75 -> [w85 w108]
          tunnel: [w84 w108] -> w74
          tunnel: [w83 w107] -> w73
          tunnel: [w82 FALSE] -> w72
          tunnel: w69 -> [w79 _]
          tunnel: w68 -> [w78 _]
          frame No Error {
            n231 = node-c288() -> (w87:T1)  [unwired: 4 in]
            n232 = timed-loop {
              tunnel: w85 -> [w101]
              tunnel: w80 -> [w100]
              tunnel: [w99] -> w84
              tunnel: [w98] -> w83
              tunnel: [w88] -> w82
              shift-right: [w92] -> _
              shift-left: FALSE -> [w95]
              timing: w87 -> [_]
              timing-out: [_] -> w86
              tunnel: w79 -> [w91]
              tunnel: w78 -> [w90]
              stop <- w96 stop-if-true
              w88 = FALSE
              n233 = node-c288() -> ()  [unwired: 1 in, 1 out]
              n234 = Dequeue Element(queue=w91, error in (no error)=w90) -> (element=w89:string)  [unwired: 1 in, 3 out]
              n235 = Select(t=FALSE, s=w95, f=TRUE) -> (s? t:f=w92:bool)
              "TCP packet\nSend To SEPTIC" <- w92
              n236 = TCP Write(connection ID=w101, data in=w89, error in (no error)=w100) -> (connection ID out=w99:refnum<k5>, error out=w98:errorcluster)  [unwired: 1 in, 1 out]
              n237 = Unbundle(w98) -> ("status"=w97:bool)  [unwired: 2 out]
              n238 = node-c288() -> ()  [unwired: 1 in, 1 out]
              n239 = Compound Arithmetic op=OR(w97, w88) -> (w96:bool)
            }
            n240 = node-c288(w86) -> ()  [unwired: 1 out]
          }
          frame Error {
          }
        }
        n241 = TCP Close Connection(connection ID=w74, error in (no error)=w73) -> (error out=→"SEPTIC TCP Error Out":errorcluster)  [unwired: 1 in, 1 out]
        n242 = Wait (ms)(milliseconds to wait=u32 1000) -> ()  [unwired: 1 out]
      }
      n243 = while {
        stop <- FALSE stop-if-true
        n244 = node-c288() -> (w371:T1)  [unwired: 4 in]
        n245 = Create Network Stream Reader Endpoint(7:10 ("reader buffer size"), 9:T4 {"Message"="", "Message Data"=variant} ("Message Cluster"), 11:"/command/reader/CO" ("reader url")) -> (0:w377:errorcluster, 3:w378:refnum<k21>)  [unwired: 4 in]
        n246 = timed-loop "Host->Target Command Reader" {
          shift-right: [w388] -> w375
          shift-left: w377 -> [w391]
          shift-right: [w389] -> w374
          shift-left: w378 -> [w390]
          tunnel: [TRUE] -> _
          timing: w371 -> [_]
          timing-out: [_] -> w370
          stop <- w382 stop-if-true
          # "Receive Commands from Host VI"
          n247 = node-c288() -> ()  [unwired: 1 in, 1 out]
          n248 = shared-variable-read(w390, w391) -> (w389:refnum<k21>, w384:errorcluster, w386:bool, w387:T4)  [unwired: 1 in]
          n249 = Or(x=w386, y=w384) -> (x .or. y?=w385:bool)
          n250 = case shown="False" w385 {
            selector: w385 -> [_ w428]
            tunnel: w384 -> [w399 w429]
            tunnel: [w398 w429] -> w388
            tunnel: w387 -> [w397 _]
            tunnel: [w394 w428] -> w382
            frame False {
              n251 = Unbundle By Name(w397) -> ("Message"=w396:string, "Message Data"=w395:variant)
              n252 = case shown="\"Flight Number\"" w396 {
                tunnel: w399 -> [w403 w408 w410 w416 w422 w427]
                tunnel: [w400 w405 w410 w415 w421 w426] -> w398
                tunnel: w395 -> [w404 w409 _ w414 w420 w425]
                tunnel: [_ _ TRUE _ _ _] -> w394
                frame "Stop File Write" {
                  n253 = Variant To Data(error in=w403, type=FALSE, Variant=w404) -> (data=→"Stop File Write":bool, error out=w400:errorcluster)
                }
                frame "Flight Number" {
                  n254 = Variant To Data(error in=w408, type="", Variant=w409) -> (data=→"Flight Number":string, error out=w405:errorcluster)
                }
                frame "Stop", Default {
                }
                frame "CO CAL" {
                  n255 = Variant To Data(error in=w416, type=FALSE, Variant=w414) -> (data=→"CO CAL":bool, error out=w415:errorcluster)
                }
                frame "CO Vacuum" {
                  n256 = Variant To Data(error in=w422, type=FALSE, Variant=w420) -> (data=w417:bool, error out=w421:errorcluster)
                  "CO Vacuum" <- w417
                  n257 = Boolean To (0,1)(Boolean=w417) -> (0, 1=→"CO Vacuum?":i16)
                  n258 = shared-variable "NI-cRIO9022-019C2C95\\Mod6\\DO5"(w417) -> ()  [unwired: 1 in, 1 out]
                }
                frame "UDP Time Offset" {
                  n259 = Variant To Data(error in=w427, type=0, Variant=w425) -> (data=→"UDP Time Stamp Offset":i32, error out=w426:errorcluster)
                }
              }
            }
            frame True {
            }
          }
          n260 = node-c288() -> ()  [unwired: 1 in, 1 out]
        }
        n261 = node-c288(w370) -> ()  [unwired: 1 out]
        n262 = Destroy Stream Endpoint(8:w375, 11:w374) -> (0:→"error out":errorcluster)
        n263 = Wait (ms)(milliseconds to wait=u32 1000) -> ()  [unwired: 1 out]
      }
      n264 = node-c288(w38) -> ()  [unwired: 1 out]
    }
    frame Error {
    }
  }
  n265 = disable-structure shown="Enabled" {
    frame Disabled {
      n266 = while {
        stop <- FALSE stop-if-true
        # "Must delay to avoid 100% CPU on cRIO"
        # "CO Control Data Loop"
        n267 = call <vilib>:"TCP Listen.vi"("port"=u16 1002) -> ("error out"=w720:errorcluster, "connection ID"=w721:refnum<k5>)  [unwired: 6 in, 3 out]
        n268 = node-c288() -> (w724:T1)  [unwired: 4 in]
        n269 = timed-loop {
          timing: w724 -> [_]
          timing-out: [_] -> w723
          tunnel: w721 -> [w741]
          tunnel: w720 -> [w740]
          tunnel: [w730] -> w719
          tunnel: [w729] -> w718
          stop <- w729 stop-if-true
          n270 = node-c288() -> ()  [unwired: 1 in, 1 out]
          n271 = TCP Read(connection ID=w741, bytes to read=4, error in (no error)=w740) -> (connection ID out=w738:refnum<k5>, data out=w735:string, error out=w737:errorcluster)  [unwired: 2 in]
          n272 = Type Cast(type=0, x=w735) -> (*(type *) &x=w734:i32)
          n273 = TCP Read(connection ID=w738, bytes to read=w734, error in (no error)=w737) -> (connection ID out=w730:refnum<k5>, data out=w731:string, error out=w729:errorcluster)  [unwired: 2 in]
          "Control data out" <- w731
          n274 = Spreadsheet String To Array(delimiter (Tab)=",", format string="%b", spreadsheet string=w731, array type (2D Dbl)=i32[] []) -> (array=w728:i32[])
          "Control data" <- w728
          n275 = Index Array(array=w728) -> (element #2=w726:i32)  [unwired: 2 in, 1 out]
          n276 = Not Equal To 0?(x=w726) -> (x != 0?=w725:bool)
          n277 = shared-variable "NI-cRIO9022-019C2C95\\Mod6\\DO5"(w725) -> ()  [unwired: 1 in, 1 out]
          n278 = node-c288() -> ()  [unwired: 1 in, 1 out]
        }
        n279 = Wait (ms)(milliseconds to wait=u32 1000) -> ()  [unwired: 1 out]
        n280 = node-c288(w723) -> ()  [unwired: 1 out]
        n281 = TCP Close Connection(connection ID=w719, error in (no error)=w718) -> ()  [unwired: 1 in, 2 out]
      }
    }
    frame Enabled {
    }
  }
  n282 = VISA Close(VISA resource name=w14, error in (no error)=w15) -> (error out=→"Serial VISA error":errorcluster)
